vi "Check Fillable.vi"(10 "Column":string, 11 "Data In":T1) -> (1 "Full?":bool, 2 "Index":i32, 3 "Fillable":bool)   [LabVIEW 2020]
uses:
  Data.ctl
panel:
  out "Array":string[][](array[string])
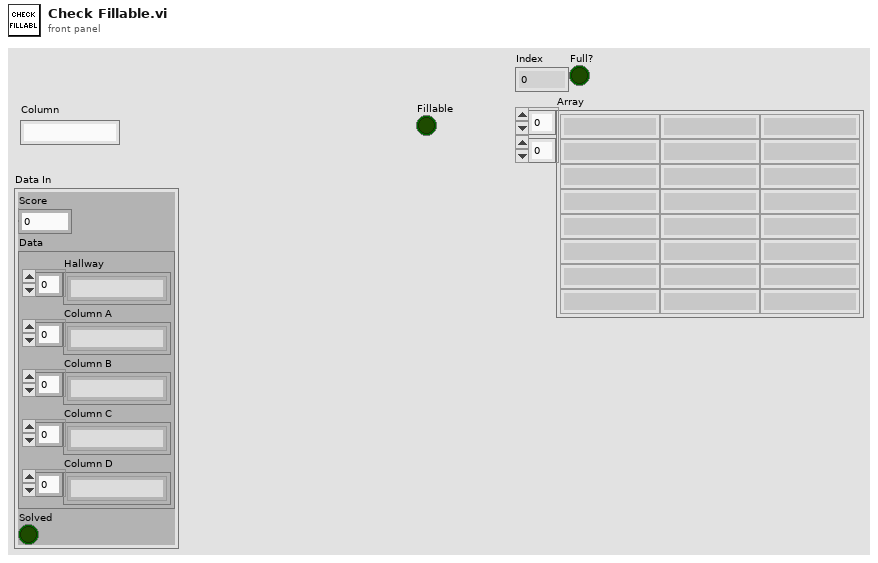
[diagram p1: front panel]
types:
  T1 = typedef "Data.ctl" = cluster{"Score":i64, "Data":cluster{"Hallway":string[], "Column A":string[], "Column B":string[], "Column C":string[], "Column D":string[]}, "Solved":bool}
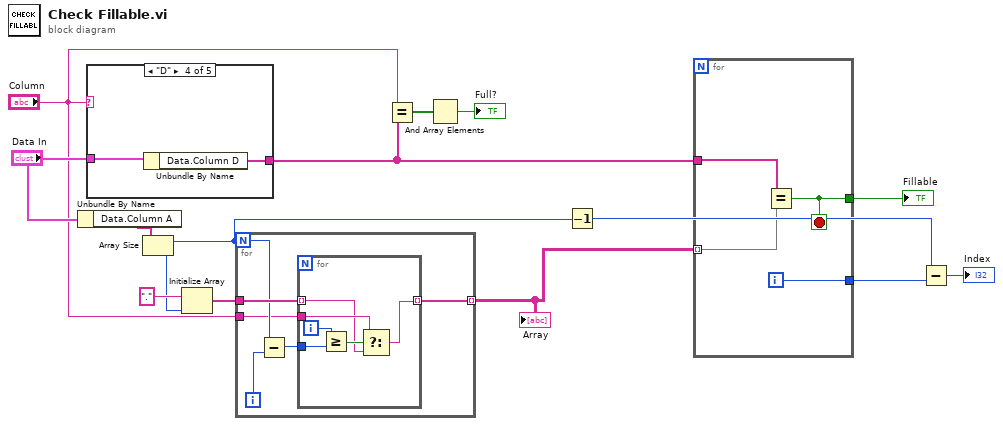
[diagram p0: block diagram]
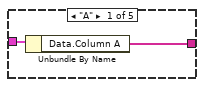
[diagram p2: hidden frame]
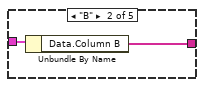
[diagram p3: hidden frame]
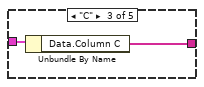
[diagram p4: hidden frame]
diagram:
  n1 = Unbundle By Name("Data In") -> ("Data.Column A"=w5:string[])
  n2 = case shown="\"D\"" "Column" {
    tunnel: "Data In" -> [w16 w18 w20 w22 _]
    tunnel: [w15 w17 w19 w21 _] -> w4
    frame "A" {
      n3 = Unbundle By Name(w16) -> ("Data.Column A"=w15:string[])
    }
    frame "B" {
      n4 = Unbundle By Name(w18) -> ("Data.Column B"=w17:string[])
    }
    frame "C" {
      n5 = Unbundle By Name(w20) -> ("Data.Column C"=w19:string[])
    }
    frame "D" {
      n6 = Unbundle By Name(w22) -> ("Data.Column D"=w21:string[])
    }
    frame Default {
    }
  }
  n7 = Array Size(array=w5) -> (size(s)=w7:i32)
  n8 = Initialize Array(".", w7) -> (w10:string[])
  n9 = for {
    N: w7 -> [w24]
    tunnel: w10 -> [w28]
    tunnel: [w27] -> w9 mode=indexing
    tunnel: "Column" -> [w23]
    i -> [w26]
    n10 = Subtract(x=w24, y=w26) -> (x-y=w25:i32)
    n11 = for {
      tunnel: w28 -> [w29] mode=indexing
      tunnel: [w30] -> w27 mode=indexing
      tunnel: w25 -> [w33]
      tunnel: w23 -> [w31]
      i -> [w34]
      n12 = Greater Or Equal?(x=w34, y=w33) -> (x >= y?=w32:bool)
      n13 = Select(t=w31, s=w32, f=w29) -> (s? t:f=w30:string)
    }
  }
  "Array" <- w9
  n14 = Equal?(x="Column", y=w4) -> (x = y?=w2:bool[])
  n15 = And Array Elements(Boolean array=w2) -> (logical AND=→"Full?":bool)
  n16 = Decrement(x=w7) -> (x-1=w6:i32)
  n17 = for {
    tunnel: w4 -> [w37]
    tunnel: w9 -> [w38] mode=indexing
    tunnel: [w36] -> w14
    tunnel: [w35] -> w13
    i -> [w35]
    stop <- w36 stop-if-true
    n18 = Equal?(x=w37, y=w38) -> (x = y?=w36:bool)
  }
  "Fillable" <- w14
  n19 = Subtract(x=w6, y=w13) -> (x-y=→"Index":i32)
